vi "Read.vi"(7 "SFTP Attributes In":refnum<class "SFTP Attributes.lvclass">, 8 "Error In":errorcluster, 10 "Max Data Length":i32=1024, 11 "SFTP Directory In":refnum<class "SFTP Directory.lvclass">) -> (0 "Error Out":errorcluster, 1 "End-of-File?":bool, 2 "Data":u8[](array[numeric]), 3 "SFTP Directory Out":refnum<class "SFTP Directory.lvclass">, 5 "SFTP Attributes Out":refnum<class "SFTP Attributes.lvclass">)   [LabVIEW 2018, in "Toolkit.lvlib" / "SFTP Directory.lvclass"]
uses:
  SFTP Directory.lvclass
  SFTP Attributes/SFTP Attributes.lvclass
  SFTP Directory.lvclass/SFTP Directory.ctl
  SFTP Attributes/SFTP Attributes.lvclass/SFTP Attributes.ctl
  Toolkit.lvlib
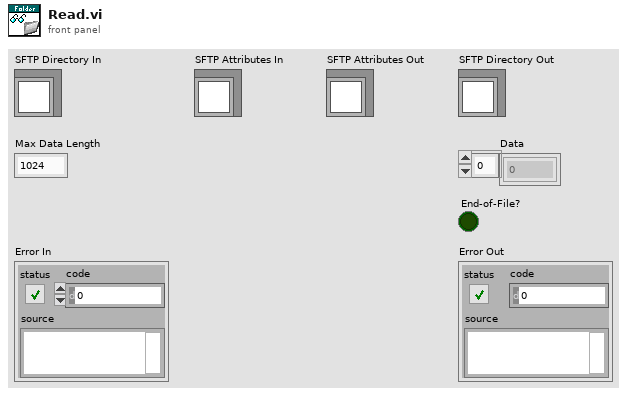
[diagram p1: front panel]
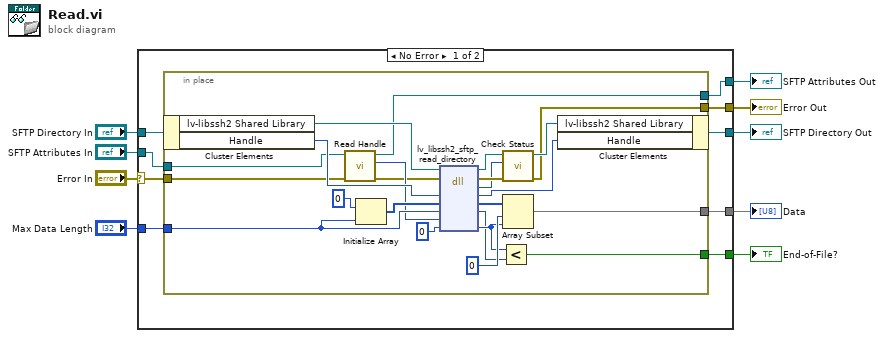
[diagram p0: block diagram]
diagram:
  n1 = case shown="No Error" "Error In" {
    selector: "Error In" -> [w17 w43]
    tunnel: "SFTP Directory In" -> [w18 w44]
    tunnel: [w16 w44] -> w3
    tunnel: [w15 w43] -> w8
    tunnel: [w14 _] -> w7
    tunnel: "Max Data Length" -> [w13 _]
    tunnel: [w12 _] -> w5
    tunnel: "SFTP Attributes In" -> [w11 w42]
    tunnel: [w10 w42] -> w1
    frame No Error {
      n2 = in-place {
        in-place-border: w17 -> [w23]
        in-place-border: [w34] -> w15
        in-place-border: [w27] -> w14
        in-place-border: w13 -> [w31]
        in-place-border: [w24] -> w12
        in-place-border: w11 -> [w22]
        in-place-border: [w19] -> w10
        n3 = in-place-cluster #1(w18) -> ("lv-libssh2 Shared Library"=w41:path, "Handle"=w40:u64)
        n4 = call "Read Handle.vi"("Error In"=w23, "SFTP Attributes In"=w22) -> ("Error Out"=w20:errorcluster, "Handle"=w21:u64, "SFTP Attributes Out"=w19:refnum<class "SFTP Attributes.lvclass">)  [unwired: 7 in]
        n5 = Initialize Array(u8 0, w31) -> (w32:u8[])
        n6 = dll-call lib="lv-libssh2.*" fn="lv_libssh2_sftp_read_directory"(path in=w41, error in=w20, "handle"=w40, "buffer"=w32, "buffer_max_length"=w31, "attributes"=w21, "read_count"=i64 0) -> (path out=w37:path, error out=w38:errorcluster, "status"=w35:i32, "handle"=w39:u64, "buffer"=w29:u8[], "buffer_max_length"=w25:u64, "read_count"=w26:i64)  [unwired: 2 in]
        n7 = Less?(x=w26, y=w25) -> (x < y?=w24:bool)
        n8 = call "Check Status.vi"("Error In"=w38, "Status"=w35, "lv-libssh2 Shared Library In"=w37) -> ("Error Out"=w34:errorcluster, "lv-libssh2 Shared Library Out"=w36:path)  [unwired: 7 in]
        n9 = Array Subset(array=w29, index=0, length=w26) -> (w27:u8[])
        n10 = in-place-cluster #1("lv-libssh2 Shared Library"=w36, "Handle"=w39) -> (w16:refnum<class "SFTP Directory.lvclass">)
      }
    }
    frame Error {
    }
  }
  "Error Out" <- w8
  "Data" <- w7
  "End-of-File?" <- w5
  "SFTP Directory Out" <- w3
  "SFTP Attributes Out" <- w1
